vi "UI.vi"(11 "Message Queues out":T1) -> ()   [LabVIEW 2024]
doc: "This UI VI which handle all UI actions"
uses:
  controls/Serial - Settings.ctl
  controls/Units.ctl
  Message Queue/All Message Queues.ctl
  Message Queue/Message Cluster.ctl
  <vilib>/Utility/miscctls.llb/LVRectTypeDef.ctl
  <vilib>/Utility/miscctls.llb/LVPointTypeDef.ctl
  <vilib>/Utility/miscctls.llb/LVPositionTypeDef.ctl
  controls/GlobalData.vi
  Message Queue/Enqueue Message (Single).vi
  Message Queue/Message Queue.lvlib
panel:
  out "Title":string
  in  "Time Array":i32[](array[numeric])
  out "Weight Raw":dbl format="%#.1f"
  out "Pressure Raw":dbl format="%#.3f"
  out "Salinity Raw":dbl format="%#.1f"
  out "Temperature Raw":dbl format="%#.1f"
  in  "Temperature Cal":T2={"C (Y-Intercept)"=0.0, "M (Gradient)"=100.0}
  in  "Pressure Cal":T2={"C (Y-Intercept)"=0.0, "M (Gradient)"=100.0}
  in  "Salinity Cal":T2={"C (Y-Intercept)"=0.0, "M (Gradient)"=100.0}
  in  "Weight Cal":T2={"C (Y-Intercept)"=0.0, "M (Gradient)"=100.0}
  in  "Tab Control":enum32{"MAIN", "settings"}(tab)
  out "Weight":dbl format="%#.1f"
  in  "Measurement Statstics":string[][](table)=[["", "", "", "", "", "", "", "", "", "", ""], ["", "", "", "", "", "", "", "", "", "", ""], ["", "", "", "", "", "", "", "", "", "", ""], ["", "", "", "", "", "", "", "", "", "", ""]]
  out "Measurement Graphs":T3
  in  "Generate Report":bool
  in  "Start recording":bool
  in  "End recording":bool
  in  "Settings Button":bool
  in  "Close Button":bool
  in  "Calibrate sensor":bool
  out "Pressure":dbl format="%#.3f"
  out "Salinity":dbl format="%#.1f"
  out "Temperature":dbl format="%#.1f"
  in  "Disable Sensor Reading":cluster{"Daq":bool, "RS232":bool}
  in  "Sampling Settings":T4={"Reading Time (ms)"=200, "Graph Time "=1000} {"Graph Time" items=["MSec"=1, "Sec"=1000]}
  in  "General Settings":T5={"Measurement Statstics"=FALSE, "Logging Type"=enum."CSV"}
  in  "Units Settings":T6={"Pressure"=enum."Pa", "Temperature"=enum."F", "Salinity"=enum."ppt", "Weight"=enum."ib"}
  in  "Weight Port Settings":T8={"Port Name"="COM1", "Port Settings"={"baud rate"=9600, "data bits"=8, "parity"=enum."None", "stop bits"=10, "flow control"=0}} {"Port Settings"."flow control" items=["None"=0, "XON/XOFF"=1, "RTS/CTS"=2, "DTR/DSR"=4]; "Port Settings"."stop bits" items=["1.0"=10, "1.5"=15, "2.0"=20]; "Port Settings"."data bits" min=5 max=8 step=1; "Port Settings"."baud rate" items=["75"=75, "110"=110, "134"=134, "150"=150, "300"=300, "600"=600, "1200"=1200, "1800"=1800, "2400"=2400, "4800"=4800, "7200"=7200, "9600"=9600, "14400"=14400, "19200"=19200, "28800"=28800, "38400"=38400, "56000"=56000, "57600"=57600, "115200"=115200, "128000"=128000, "230400"=230400]}
  in  "Channels Settings":T9={"Pressure"={"Physical Channel"="Dev1/ai0", "Min Voltage"=0.0, "Max Voltage "=10.0, "Terminal Configuration"=10083}, "Temperature"={"Physical Channel"="Dev1/ai0", "Min Current (mA)"=0.0, "Max Current (mA)"=10.0, "Terminal Configuration"=10083}, "Sallinity"={"Physical Channel"="Dev1/ai0", "Min Current (mA)"=0.0, "Max Current (mA)"=10.0, "Terminal Configuration"=10083}} {"Sallinity"."Terminal Configuration" items=["default"=-1, "RSE"=10083, "NRSE"=10078, "Differential"=10106, "Pseudodifferential"=12529]; "Temperature"."Terminal Configuration" items=["default"=-1, "RSE"=10083, "NRSE"=10078, "Differential"=10106, "Pseudodifferential"=12529]; "Pressure"."Terminal Configuration" items=["default"=-1, "RSE"=10083, "NRSE"=10078, "Differential"=10106, "Pseudodifferential"=12529]}
  in  "Back to main":bool
  in  "Save settings":bool
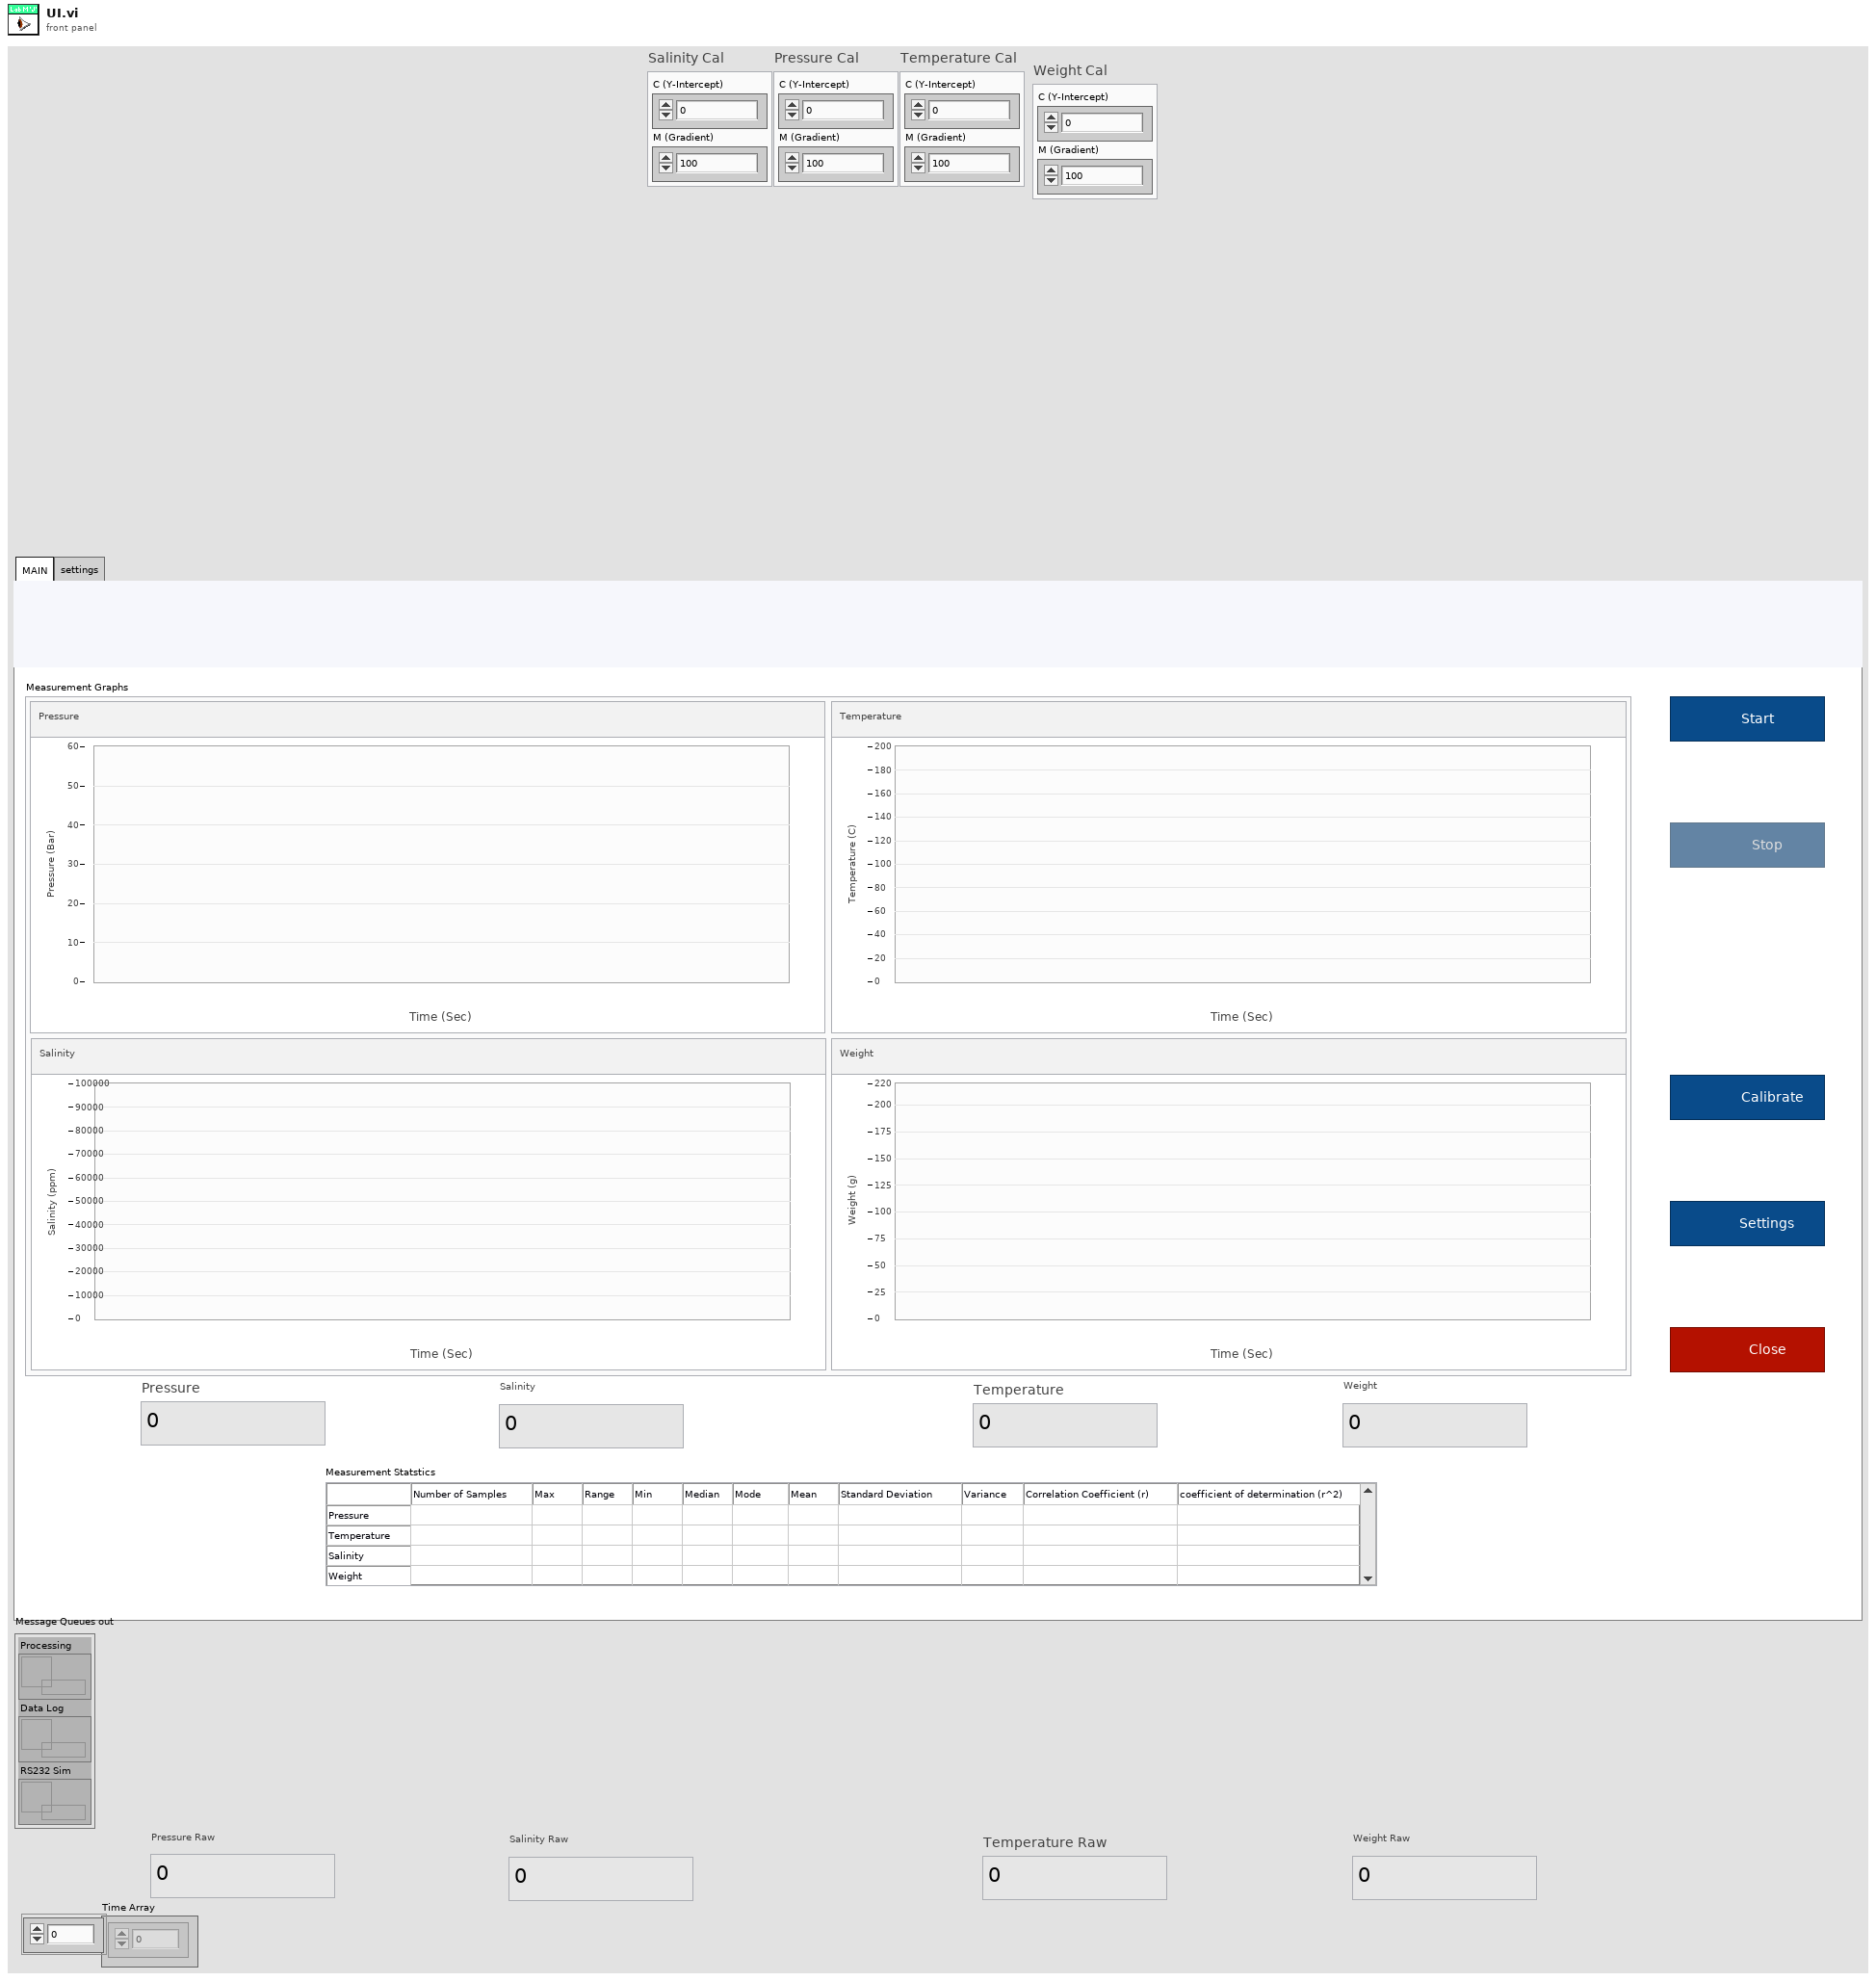
[diagram p1: front panel]
types:
  T1 = typedef "Message Queue.lvlib/All Message Queues.ctl" = cluster{"Processing":refnum<queue>, "Data Log":refnum<queue>, "RS232 Sim":refnum<queue>}
  T2 = cluster{"C (Y-Intercept)":dbl, "M (Gradient)":dbl}
  T3 = cluster{"Pressure":dbl[], "Temperature":dbl[], "Salinity":dbl[], "Weight":dbl[]}
  T4 = cluster{"Reading Time (ms)":u64, "Graph Time ":u16}
  T5 = cluster{"Measurement Statstics":bool, "Logging Type":enum16{"Disable Log", "TDMS", "CSV"}}
  T6 = typedef "Units.ctl" = cluster{"Pressure":enum16{"PSI", "Bar", "atm", "Pa"}, "Temperature":enum16{"C", "K", "F"}, "Salinity":enum16{"ppm", "ppt", "PSU"}, "Weight":enum16{"Kg", "g", "oz", "ib"}}
  T7 = typedef "Serial - Settings.ctl" = cluster{"baud rate":u32, "data bits":u16, "parity":enum16{"None", "Odd", "Even", "Mark", "Space"}, "stop bits":u16, "flow control":u16}
  T8 = cluster{"Port Name":refnum<visa-resource-name>, "Port Settings":T7}
  T9 = cluster{"Pressure":cluster{"Physical Channel":tag, "Min Voltage":dbl, "Max Voltage ":dbl, "Terminal Configuration":i32}, "Temperature":cluster{"Physical Channel":tag, "Min Current (mA)":dbl, "Max Current (mA)":dbl, "Terminal Configuration":i32}, "Sallinity":cluster{"Physical Channel":tag, "Min Current (mA)":dbl, "Max Current (mA)":dbl, "Terminal Configuration":i32}}
  T10 = typedef "LVPointTypeDef.ctl" = cluster{"Horizontal":i16, "Vertical":i16}
  T11 = typedef "LVRectTypeDef.ctl" = cluster{"Left":i16, "Top":i16, "Right":i16, "Bottom":i16}
  T12 = enum32{"Invalid", "Default", "Floating", "Floating/Auto-Hide", "Modal"}
  T13 = typedef "LVPositionTypeDef.ctl" = cluster{"Left":i32, "Top":i32}
  T14 = enum8{"Enabled", "Disabled", "Disabled and Grayed Out"}
  T15 = typedef "GlobalData.ctl" = cluster{"Measurements":cluster{"Measurement Graphs":refnum<vi>, "Pressure":refnum<vi>, "Temperature":refnum<vi>, "Salinity":refnum<vi>, "Weight":refnum<vi>, "Pressure Raw":refnum<vi>, "Temperature Raw":refnum<vi>, "Salinity Raw":refnum<vi>, "Weight Raw":refnum<vi>, "Measurement Statstics":refnum<vi>, "Time Array":refnum<vi>}, "Settings":cluster{"Sampling Settings":refnum<vi>, "General Settings":refnum<vi>, "Disable Sensor Reading":refnum<vi>, "Units Settings":refnum<vi>, "Channels Settings":refnum<vi>, "Weight Port Settings":refnum<vi>}, "Calibration Data":cluster{"Pressure Cal":refnum<vi>, "Temperature Cal":refnum<vi>, "Salinity Cal":refnum<vi>, "Weight Cal":refnum<vi>}, "UI":cluster{"Generate Report":refnum<vi>}}
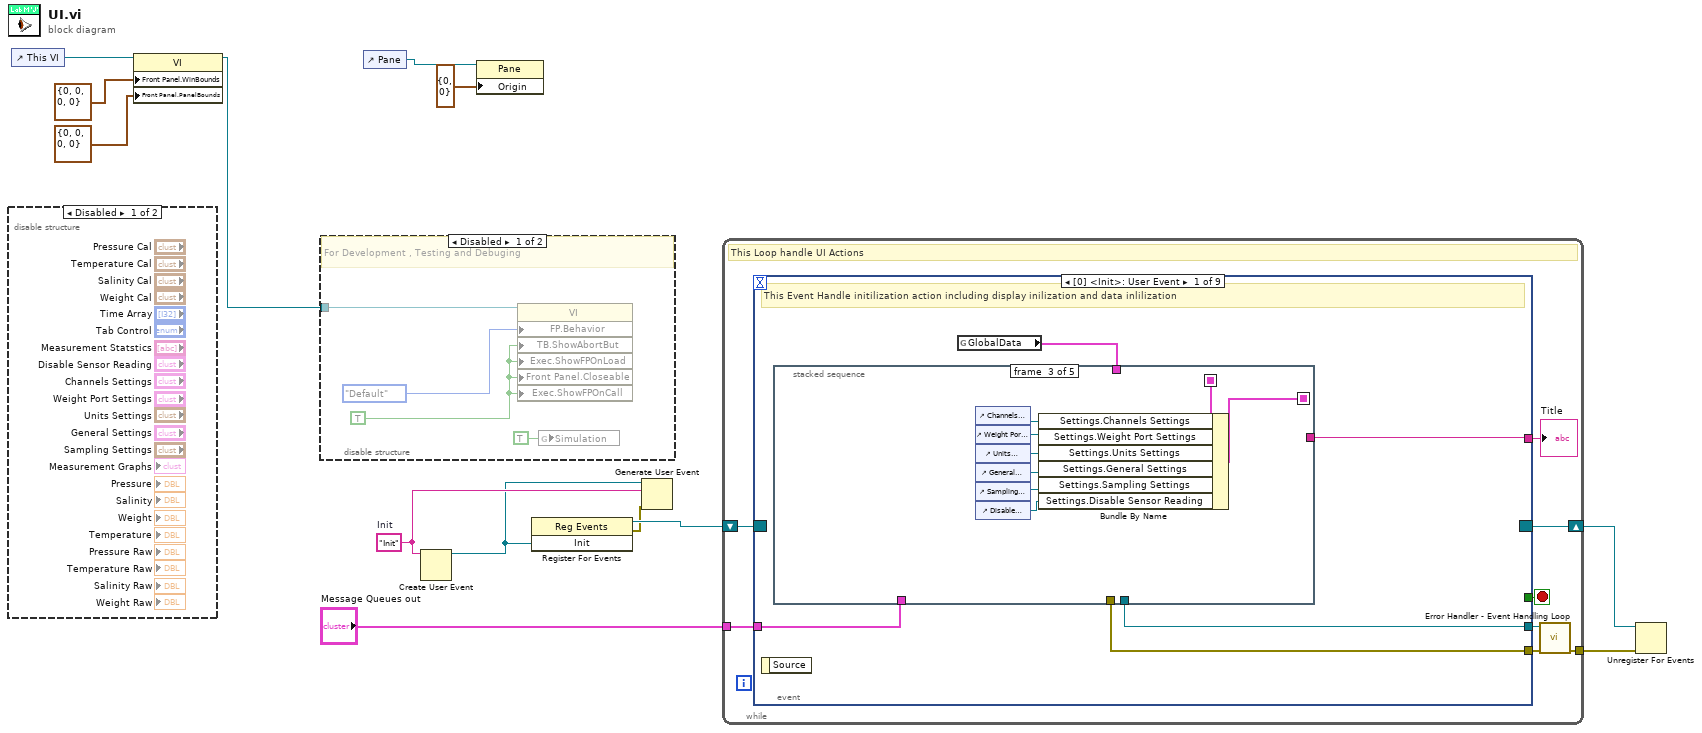
[diagram p0: block diagram]
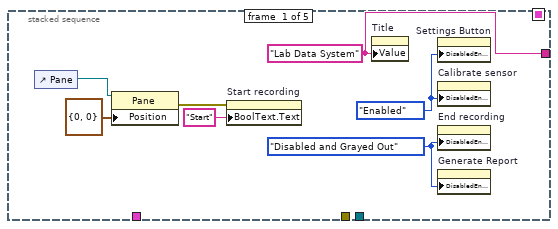
[diagram p4: hidden frame]
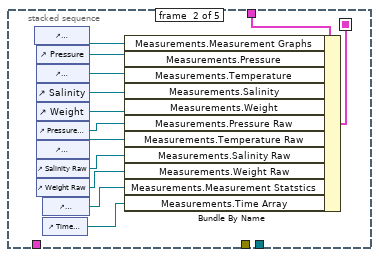
[diagram p5: hidden frame]
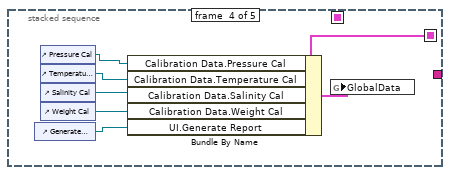
[diagram p6: hidden frame]
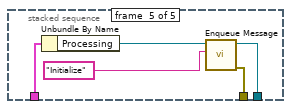
[diagram p7: hidden frame]
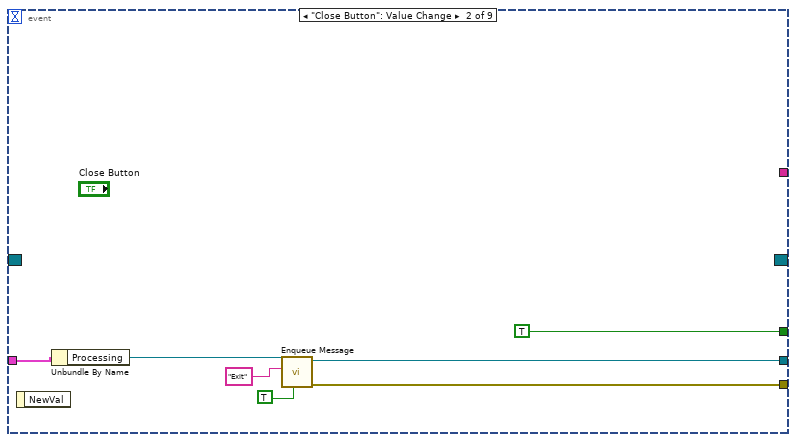
[diagram p8: hidden frame]
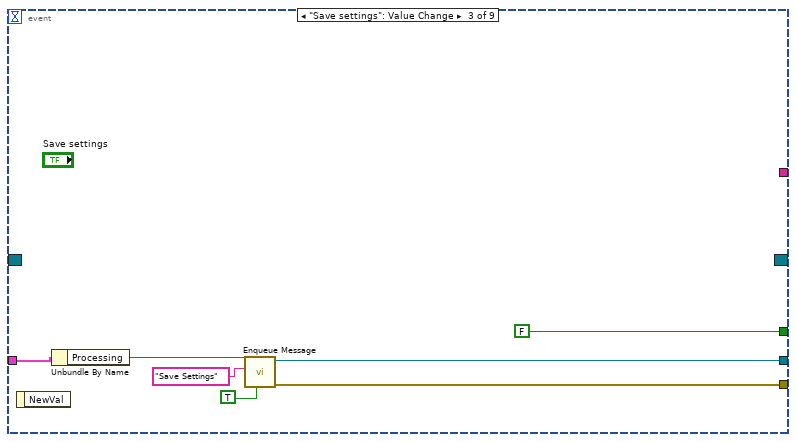
[diagram p9: hidden frame]
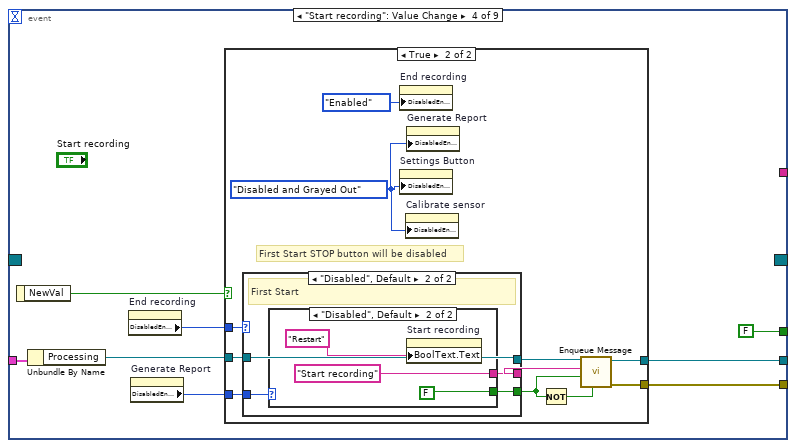
[diagram p10: hidden frame]
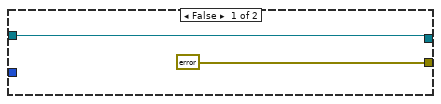
[diagram p11: hidden frame]
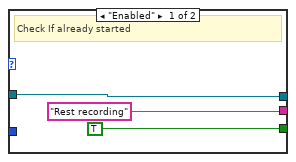
[diagram p12: hidden frame]
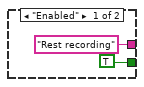
[diagram p13: hidden frame]
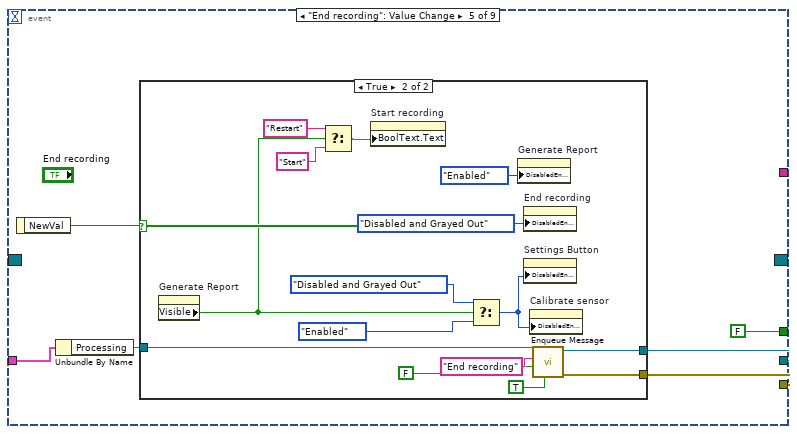
[diagram p14: hidden frame]
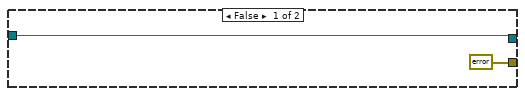
[diagram p15: hidden frame]
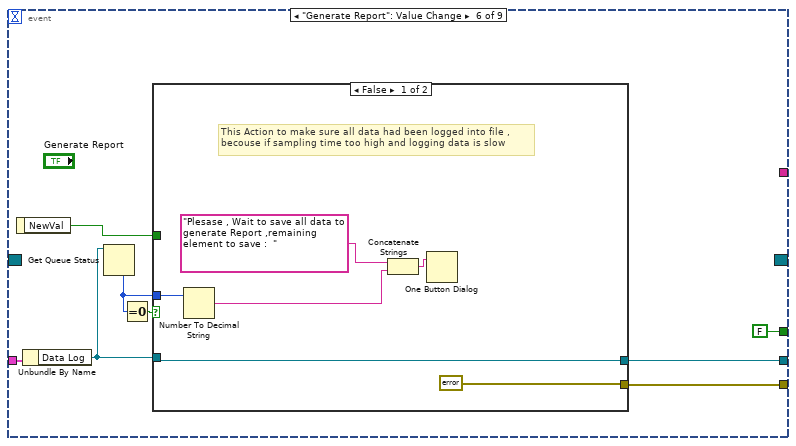
[diagram p16: hidden frame]
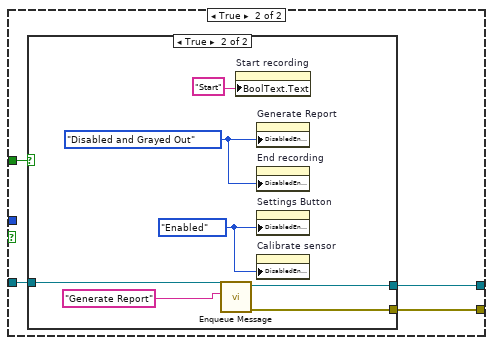
[diagram p17: hidden frame]
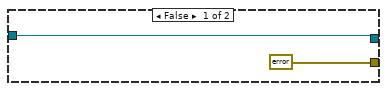
[diagram p18: hidden frame]
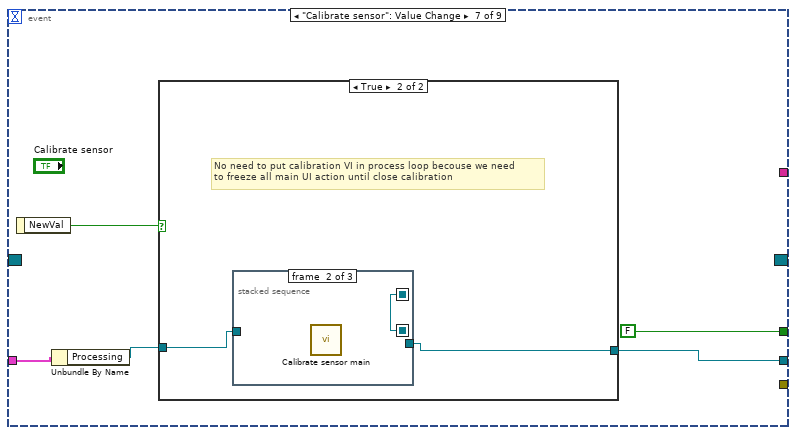
[diagram p19: hidden frame]
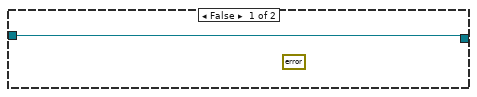
[diagram p20: hidden frame]
diagram:
  w10 = "Init"  # Init
  n1 = disable-structure shown="Disabled" {
    frame Disabled {
    }
    frame Enabled {
    }
  }
  n2 = control-ref of="This VI"() -> (w4:refnum<vi>)
  n3 = property class="VI"(reference=w4, "Front Panel.WinBounds"=T11 {"Left"=0, "Top"=0, "Right"=0, "Bottom"=0} ("Front Panel Window:Window Bounds"), "Front Panel.PanelBounds"=T11 {"Left"=0, "Top"=0, "Right"=0, "Bottom"=0} ("Front Panel Window:Panel Bounds")) -> (reference out=w5:refnum<vi>)  [unwired: 1 in, 1 out]
  n4 = disable-structure shown="Disabled" {
    disable-tunnel: w5 -> [w14 _]
    frame Disabled {
      w16 = TRUE ("Tool Bar:Show Abort Button")
      # "For Development , Testing and Debuging"
      n5 = property class="VI"(reference=w14, "FP.Behavior"=T12."Default" ("Front Panel Window:Behavior"), "TB.ShowAbortBut"=w16, "Exec.ShowFPOnLoad"=w16, "Front Panel.Closeable"=w16, "Exec.ShowFPOnCall"=w16) -> ()  [unwired: 1 in, 2 out]
      n6 = global write "GlobalData.vi" "Simulation"(TRUE ("Simulation")) -> ()
    }
    frame Enabled {
    }
  }
  n7 = control-ref of="Pane"() -> (w2:refnum<vi>)
  n8 = Create User Event(user event datatype=w10) -> (user event=w8:refnum<user-event>)  [unwired: 1 in, 1 out]
  n9 = property class="Pane"(reference=w2, "Origin"=T10 {"Horizontal"=0, "Vertical"=0}) -> ()  [unwired: 1 in, 2 out]
  n10 = register-events(w8) -> (reference out=w11:refnum<event-registration>, error out=w9:errorcluster)  [unwired: 2 in]
  n11 = Generate User Event(user event=w8, event data cluster=w10, error in=w9) -> ()  [unwired: 1 in, 2 out]
  n12 = while {
    tunnel: "Message Queues out" -> [w25]
    shift-right: [w23] -> w13
    shift-left: w11 -> [w24]
    tunnel: [w19] -> w12
    stop <- w21 stop-if-true
    # "This Loop handle UI Actions"
    n13 = event shown="[0] <Init>: User Event" {
      selector: w24 -> [_ _ _ _ _ _ _ _ _]
      dyn-events: [_ _ _ _ _ _ _ _ _] -> w23
      timeout: _ -> [_ _ _ _ _ _ _ _ _]
      tunnel: [_ TRUE ("Discard?") FALSE ("Discard?") FALSE ("Discard?") FALSE ("Discard?") FALSE ("Discard?") FALSE ("Discard?") _ _] -> w21
      tunnel: w25 -> [w30 w72 w79 w89 w120 w145 w170 w187 w190]
      tunnel: [w29 w77 w84 w92 w123 w148 _ _ _] -> w22
      tunnel: [w28 w76 w83 w91 w122 w147 w172 w186 w189] -> w20
      tunnel: [w26 _ _ _ _ _ _ "Settings" ("Title") _] -> w18
      event User Event {
        # "This Event Handle initilization action including display inilization and data inlilization"
        n14 = event-data() -> ()  [unwired: 1 in, 1 out]
        n15 = global read "GlobalData.vi" "GlobalData"() -> (w27:T15)
        n16 = stacked-sequence {
          seq-local: [_ w44 _ _ _] -> [_ _ w58 _ _]
          seq-local: [_ _ w57 _ _] -> [_ _ _ w65 _]
          tunnel: w27 -> [_ w45 _ _ _]
          tunnel: w30 -> [_ _ _ _ w69]
          tunnel: [_ _ _ _ w67] -> w29
          tunnel: [_ _ _ _ w66] -> w28
          tunnel: [w31 _ _ _ _] -> w26
          frame #0 {
            w31 = "Lab Data System" ("Title")
            w37 = T14."Enabled" ("Disabled")
            w36 = T14."Disabled and Grayed Out" ("Disabled")
            n17 = control-ref of="Pane"() -> (w35:refnum<vi>)
            n18 = property class="Pane"(reference=w35, "Position"=T13 {"Left"=0, "Top"=0}) -> (error out=w32:errorcluster)  [unwired: 1 in, 1 out]
            n19 = property on="Start recording" class="Bool"(error in=w32, "BoolText.Text"="Start" ("Boolean Text.Text")) -> ()  [unwired: 1 in, 2 out]
            n20 = property on="Title" class="Str"("Value"=w31) -> ()  [unwired: 2 in, 2 out]
            n21 = property on="Settings Button" class="Bool"("DisabledEnum"=w37) -> ()  [unwired: 2 in, 2 out]
            n22 = property on="Calibrate sensor" class="Bool"("DisabledEnum"=w37) -> ()  [unwired: 2 in, 2 out]
            n23 = property on="End recording" class="Bool"("DisabledEnum"=w36) -> ()  [unwired: 2 in, 2 out]
            n24 = property on="Generate Report" class="Bool"("DisabledEnum"=w36) -> ()  [unwired: 2 in, 2 out]
          }
          frame #1 {
            n25 = control-ref of="Measurement Graphs"() -> (w50:refnum<vi>)
            n26 = control-ref of="Pressure"() -> (w49:refnum<vi>)
            n27 = control-ref of="Temperature"() -> (w48:refnum<vi>)
            n28 = control-ref of="Salinity"() -> (w47:refnum<vi>)
            n29 = control-ref of="Weight"() -> (w46:refnum<vi>)
            n30 = control-ref of="Pressure Raw"() -> (w43:refnum<vi>)
            n31 = control-ref of="Temperature Raw"() -> (w42:refnum<vi>)
            n32 = control-ref of="Salinity Raw"() -> (w41:refnum<vi>)
            n33 = control-ref of="Weight Raw"() -> (w40:refnum<vi>)
            n34 = control-ref of="Measurement Statstics"() -> (w39:refnum<vi>)
            n35 = control-ref of="Time Array"() -> (w38:refnum<vi>)
            n36 = Bundle By Name(cluster=w45, "Measurements.Measurement Graphs"=w50, "Measurements.Pressure"=w49, "Measurements.Temperature"=w48, "Measurements.Salinity"=w47, "Measurements.Weight"=w46, "Measurements.Pressure Raw"=w43, "Measurements.Temperature Raw"=w42, "Measurements.Salinity Raw"=w41, "Measurements.Weight Raw"=w40, "Measurements.Measurement Statstics"=w39, "Measurements.Time Array"=w38) -> (w44:T15)
          }
          frame #2 {
            n37 = control-ref of="Channels Settings"() -> (w56:refnum<vi>)
            n38 = control-ref of="Weight Port Settings"() -> (w55:refnum<vi>)
            n39 = control-ref of="Units Settings"() -> (w54:refnum<vi>)
            n40 = control-ref of="General Settings"() -> (w53:refnum<vi>)
            n41 = control-ref of="Sampling Settings"() -> (w52:refnum<vi>)
            n42 = control-ref of="Disable Sensor Reading"() -> (w51:refnum<vi>)
            n43 = Bundle By Name(cluster=w58, "Settings.Channels Settings"=w56, "Settings.Weight Port Settings"=w55, "Settings.Units Settings"=w54, "Settings.General Settings"=w53, "Settings.Sampling Settings"=w52, "Settings.Disable Sensor Reading"=w51) -> (w57:T15)
          }
          frame #3 {
            n44 = control-ref of="Generate Report"() -> (w59:refnum<vi>)
            n45 = control-ref of="Pressure Cal"() -> (w64:refnum<vi>)
            n46 = control-ref of="Temperature Cal"() -> (w63:refnum<vi>)
            n47 = control-ref of="Salinity Cal"() -> (w62:refnum<vi>)
            n48 = control-ref of="Weight Cal"() -> (w61:refnum<vi>)
            n49 = Bundle By Name(cluster=w65, "Calibration Data.Pressure Cal"=w64, "Calibration Data.Temperature Cal"=w63, "Calibration Data.Salinity Cal"=w62, "Calibration Data.Weight Cal"=w61, "UI.Generate Report"=w59) -> (w60:T15)
            n50 = global write "GlobalData.vi" "GlobalData"(w60) -> ()
          }
          frame #4 {
            n51 = Unbundle By Name(w69) -> ("Processing"=w70:refnum<queue>)
            n52 = call-poly "Enqueue Message.vi"("Message"="Initialize", "Message Queue"=w70) -> ("error out"=w67:errorcluster, "dup Message Queue"=w66:refnum<queue>)  [unwired: 8 in]
          }
        }
      }
      event "Close Button": Value Change {
        n53 = event-data() -> ()  [unwired: 1 in, 1 out]
        n54 = Unbundle By Name(w72) -> ("Processing"=w71:refnum<queue>)
        n55 = call-poly "Enqueue Message.vi"("Priority Message? (F)"=TRUE, "Message"="Exit", "Message Queue"=w71) -> ("error out"=w77:errorcluster, "dup Message Queue"=w76:refnum<queue>)  [unwired: 7 in]
      }
      event "Save settings": Value Change {
        n56 = event-data() -> ()  [unwired: 1 in, 1 out]
        n57 = Unbundle By Name(w79) -> ("Processing"=w78:refnum<queue>)
        n58 = call-poly "Enqueue Message.vi"("Priority Message? (F)"=TRUE, "Message"="Save Settings", "Message Queue"=w78) -> ("error out"=w84:errorcluster, "dup Message Queue"=w83:refnum<queue>)  [unwired: 7 in]
      }
      event "Start recording": Value Change {
        n59 = event-data() -> ("NewVal"=w87:bool)  [unwired: 1 in]
        n60 = Unbundle By Name(w89) -> ("Processing"=w88:refnum<queue>)
        n61 = property on="End recording" class="Bool"() -> ("DisabledEnum"=w86:T14)  [unwired: 2 in, 2 out]
        n62 = property on="Generate Report" class="Bool"() -> ("DisabledEnum"=w85:T14)  [unwired: 2 in, 2 out]
        n63 = case shown="True" w87 {
          tunnel: [errorcluster {"status"=FALSE, "code"=0, "source"=""} ("error out") w105] -> w92
          tunnel: [w94 w104] -> w91
          tunnel: w88 -> [w94 w102]
          tunnel: w86 -> [_ w97]
          tunnel: w85 -> [_ w96]
          frame False {
          }
          frame True {
            w95 = T14."Disabled and Grayed Out" ("Disabled")
            # "First Start STOP button will be disabled"
            n64 = case shown="\"Disabled\", Default" w97 {
              tunnel: w102 -> [w108 w112]
              tunnel: [w108 w112] -> w101
              tunnel: ["Rest recording" ("Message") w111] -> w100
              tunnel: [TRUE ("Discard?") w110] -> w99
              tunnel: w96 -> [_ w109]
              frame "Enabled" {
                # "Check If already started"
              }
              frame "Disabled", Default {
                # "First Start"
                n65 = case shown="\"Disabled\", Default" w109 {
                  tunnel: ["Rest recording" ("Message") "Start recording" ("Message")] -> w111
                  tunnel: [TRUE ("Discard?") FALSE ("Discard?")] -> w110
                  frame "Enabled" {
                  }
                  frame "Disabled", Default {
                    n66 = property on="Start recording" class="Bool"("BoolText.Text"="Restart" ("Boolean Text.Text")) -> ()  [unwired: 2 in, 2 out]
                  }
                }
              }
            }
            n67 = property on="End recording" class="Bool"("DisabledEnum"=T14."Enabled" ("Disabled")) -> ()  [unwired: 2 in, 2 out]
            n68 = property on="Settings Button" class="Bool"("DisabledEnum"=w95) -> ()  [unwired: 2 in, 2 out]
            n69 = property on="Calibrate sensor" class="Bool"("DisabledEnum"=w95) -> ()  [unwired: 2 in, 2 out]
            n70 = property on="Generate Report" class="Bool"("DisabledEnum"=w95) -> ()  [unwired: 2 in, 2 out]
            n71 = Not(x=w99) -> (.not. x?=w98:bool)
            n72 = call-poly "Enqueue Message.vi"("Priority Message? (F)"=w98, "Message Data"=w99, "Message"=w100, "Message Queue"=w101) -> ("error out"=w105:errorcluster, "dup Message Queue"=w104:refnum<queue>)  [unwired: 6 in]
          }
        }
      }
      event "End recording": Value Change {
        n73 = event-data() -> ("NewVal"=w118:bool)  [unwired: 1 in]
        n74 = Unbundle By Name(w120) -> ("Processing"=w119:refnum<queue>)
        n75 = case shown="True" w118 {
          tunnel: [errorcluster {"status"=FALSE, "code"=0, "source"=""} ("error out") w140] -> w123
          tunnel: [w125 w139] -> w122
          tunnel: w119 -> [w125 w137]
          frame False {
          }
          frame True {
            n76 = property on="Generate Report" class="Bool"() -> ("Visible"=w128:bool)  [unwired: 2 in, 2 out]
            n77 = Select(t="Restart", s=w128, f="Start" ("Boolean Text.Text")) -> (s? t:f=w130:string)
            n78 = property on="Start recording" class="Bool"("BoolText.Text"=w130) -> ()  [unwired: 2 in, 2 out]
            n79 = Select(t=T14."Disabled and Grayed Out" ("Disabled"), s=w128, f=T14."Enabled" ("Disabled")) -> (s? t:f=w131:T14)
            n80 = property on="Generate Report" class="Bool"("DisabledEnum"=T14."Enabled" ("Disabled")) -> ()  [unwired: 2 in, 2 out]
            n81 = property on="End recording" class="Bool"("DisabledEnum"=T14."Disabled and Grayed Out" ("Disabled")) -> ()  [unwired: 2 in, 2 out]
            n82 = property on="Settings Button" class="Bool"("DisabledEnum"=w131) -> ()  [unwired: 2 in, 2 out]
            n83 = property on="Calibrate sensor" class="Bool"("DisabledEnum"=w131) -> ()  [unwired: 2 in, 2 out]
            n84 = call-poly "Enqueue Message.vi"("Priority Message? (F)"=TRUE, "Message Data"=FALSE ("Priority Message? (F)"), "Message"="End recording", "Message Queue"=w137) -> ("error out"=w140:errorcluster, "dup Message Queue"=w139:refnum<queue>)  [unwired: 6 in]
          }
        }
      }
      event "Generate Report": Value Change {
        n85 = event-data() -> ("NewVal"=w144:bool)  [unwired: 1 in]
        n86 = Unbundle By Name(w145) -> ("Data Log"=w143:refnum<queue>)
        n87 = Get Queue Status(queue=w143) -> (# elements in queue=w141:i32)  [unwired: 2 in, 7 out]
        n88 = Equal To 0?(x=w141) -> (x = 0?=w142:bool)
        n89 = case shown="False" w142 {
          tunnel: [errorcluster {"status"=FALSE, "code"=0, "source"=""} ("error out") w158] -> w148
          tunnel: [w150 w157] -> w147
          tunnel: w143 -> [w150 w156]
          tunnel: w144 -> [_ w155]
          tunnel: w141 -> [w153 _]
          frame False {
            # "This Action to make sure all data had been logged into file ,\nbecouse if sampling time too high and logging data is slow"
            n90 = Number To Decimal String(number=w153) -> (decimal integer string=w152:string)  [unwired: 1 in]
            n91 = Concatenate Strings("Plesase , Wait to save all data to generate Report ,remaining element to save :  " ("string"), w152) -> (w151:string)
            n92 = One Button Dialog(message=w151) -> ()  [unwired: 1 in, 1 out]
          }
          frame True {
            n93 = case shown="True" w155 {
              tunnel: [errorcluster {"status"=FALSE, "code"=0, "source"=""} ("error out") w167] -> w158
              tunnel: [w160 w166] -> w157
              tunnel: w156 -> [w160 w164]
              frame False {
              }
              frame True {
                w163 = T14."Disabled and Grayed Out" ("Disabled")
                w162 = T14."Enabled" ("Disabled")
                n94 = call-poly "Enqueue Message.vi"("Message"="Generate Report", "Message Queue"=w164) -> ("error out"=w167:errorcluster, "dup Message Queue"=w166:refnum<queue>)  [unwired: 8 in]
                n95 = property on="Start recording" class="Bool"("BoolText.Text"="Start" ("Boolean Text.Text")) -> ()  [unwired: 2 in, 2 out]
                n96 = property on="Generate Report" class="Bool"("DisabledEnum"=w163) -> ()  [unwired: 2 in, 2 out]
                n97 = property on="End recording" class="Bool"("DisabledEnum"=w163) -> ()  [unwired: 2 in, 2 out]
                n98 = property on="Settings Button" class="Bool"("DisabledEnum"=w162) -> ()  [unwired: 2 in, 2 out]
                n99 = property on="Calibrate sensor" class="Bool"("DisabledEnum"=w162) -> ()  [unwired: 2 in, 2 out]
              }
            }
          }
        }
      }
      event "Calibrate sensor": Value Change {
        n100 = event-data() -> ("NewVal"=w168:bool)  [unwired: 1 in]
        n101 = Unbundle By Name(w170) -> ("Processing"=w169:refnum<queue>)
        n102 = case shown="True" w168 {
          tunnel: [w173 w174] -> w172
          tunnel: w169 -> [w173 w175]
          frame False {
            (unwired) errorcluster {"status"=FALSE, "code"=0, "source"=""} ("error out")
          }
          frame True {
            # "No need to put calibration VI in process loop becouse we need\nto freeze all main UI action until close calibration"
            n103 = stacked-sequence {
              seq-local: [w178 _ _] -> [_ w180 _]
              seq-local: [_ w180 _] -> [_ _ w183]
              tunnel: w175 -> [w179 _ _]
              tunnel: [_ _ w182] -> w174
              frame #0 {
                n104 = call-poly "Enqueue Message.vi"("Message Data"=TRUE ("Discard?"), "Message"="Start recording", "Message Queue"=w179) -> ("dup Message Queue"=w178:refnum<queue>)  [unwired: 7 in, 1 out]
              }
              frame #1 {
                n105 = call "Calibrate sensor main.vi"() -> ()  [unwired: 12 in]
              }
              frame #2 {
                w181 = TRUE ("Priority Message? (F)")
                n106 = call-poly "Enqueue Message.vi"("Priority Message? (F)"=w181, "Message Data"=w181, "Message"="End recording", "Message Queue"=w183) -> ("dup Message Queue"=w182:refnum<queue>)  [unwired: 6 in, 1 out]
              }
            }
          }
        }
      }
      event "Settings Button": Value Change {
        n107 = event-data() -> ()  [unwired: 1 in, 6 out]
        n108 = Unbundle By Name(w187) -> ("Processing"=w186:refnum<queue>)
        n109 = property on="Tab Control" class="TabCtl (strict)"("Value"=enum32{"MAIN", "settings", "About"}."settings" ("Tab Control")) -> ()  [unwired: 2 in, 2 out]
      }
      event "Back to main": Value Change {
        n110 = event-data() -> ()  [unwired: 1 in, 6 out]
        n111 = Unbundle By Name(w190) -> ("Processing"=w189:refnum<queue>)
        n112 = property on="Tab Control" class="TabCtl (strict)"("Value"=enum32{"MAIN", "settings", "About"}."MAIN" ("Tab Control")) -> ()  [unwired: 2 in, 2 out]
      }
    }
    "Title" <- w18
    n113 = call "Error Handler - Event Handling Loop.vi"("error in (no error)"=w22, "Message Queue"=w20) -> ("dup error in"=w19:errorcluster)  [unwired: 8 in, 1 out]
  }
  n114 = Unregister For Events(event registration refnum=w13, error in=w12) -> ()  [unwired: 1 out]
